vi "Deadband.vi"(10 "Deadband":dbl, 11 "Motor Speed":dbl) -> (3 "Power Out":dbl)   [LabVIEW 2014]
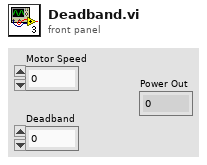
[diagram p1: front panel]
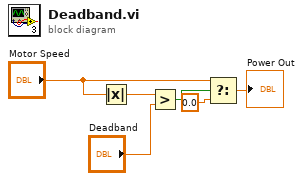
[diagram p0: block diagram]
diagram:
  n1 = Absolute Value(x="Motor Speed") -> (abs(x)=w6:dbl)
  n2 = Greater?(x=w6, y="Deadband") -> (0:w4:bool)
  n3 = Select(t="Motor Speed", s=w4, f=0.0) -> (s? t:f=→"Power Out":dbl)
